vi "ChangePlotSize.vi"(8 "error in (no error)":errorcluster caption="错误输入（无错误）", 11 "TPlot 输入":refnum<class "TPlot.lvclass">) -> (0 "error out":errorcluster caption="错误输出", 3 "TPlot 输出":refnum<class "TPlot.lvclass">)   [LabVIEW 2018, in "DataDisplay.lvlib" / "TPlot.lvclass"]
uses:
  TPlot.lvclass
  <vilib>/Utility/miscctls.llb/LVBoundsTypeDef.ctl
  <vilib>/Utility/miscctls.llb/LVPositionTypeDef.ctl
  TPlot.lvclass/TPlot.ctl
panel:
  out "波形图":waveform(dbl)[](graph)
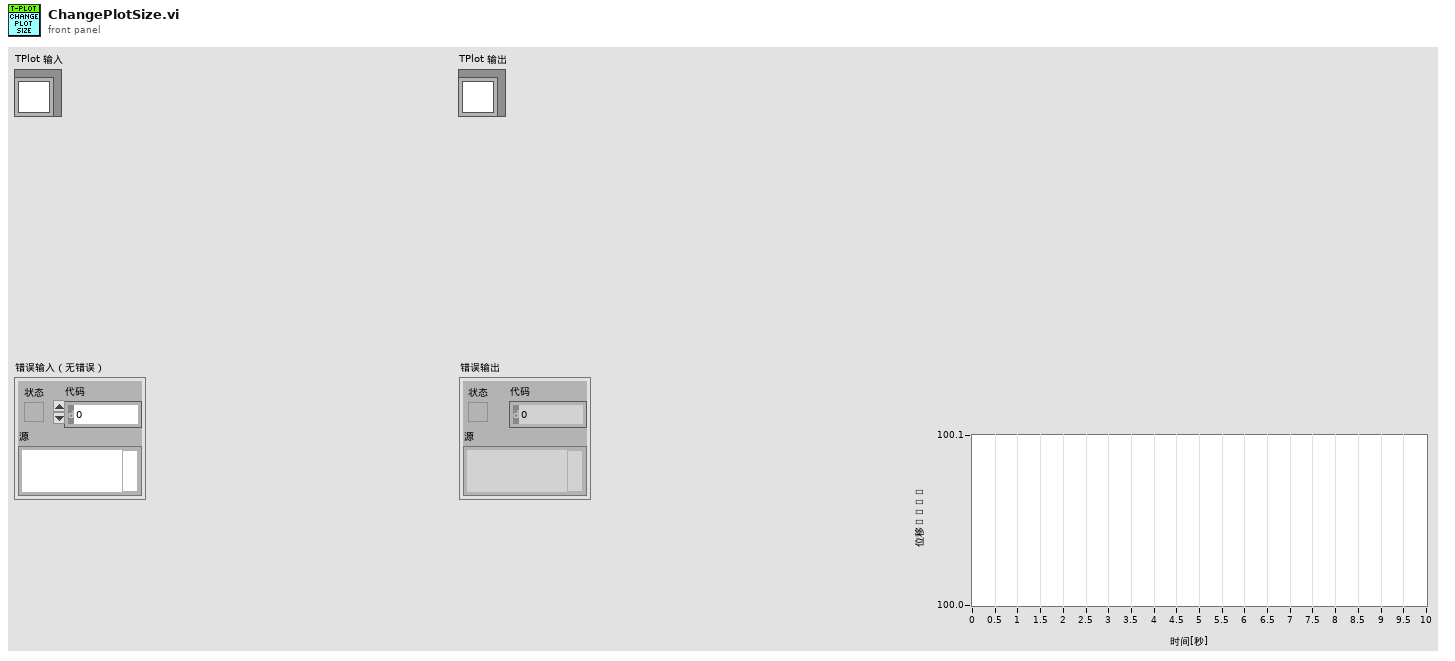
[diagram p1: front panel]
types:
  T1 = typedef "LVPositionTypeDef.ctl" = cluster{"Left":i32, "Top":i32}
  T2 = typedef "LVBoundsTypeDef.ctl" = cluster{"Width":u32, "Height":u32}
  T3 = typedef "LVRectTypeDef.ctl" = cluster{"Left":i16, "Top":i16, "Right":i16, "Bottom":i16}
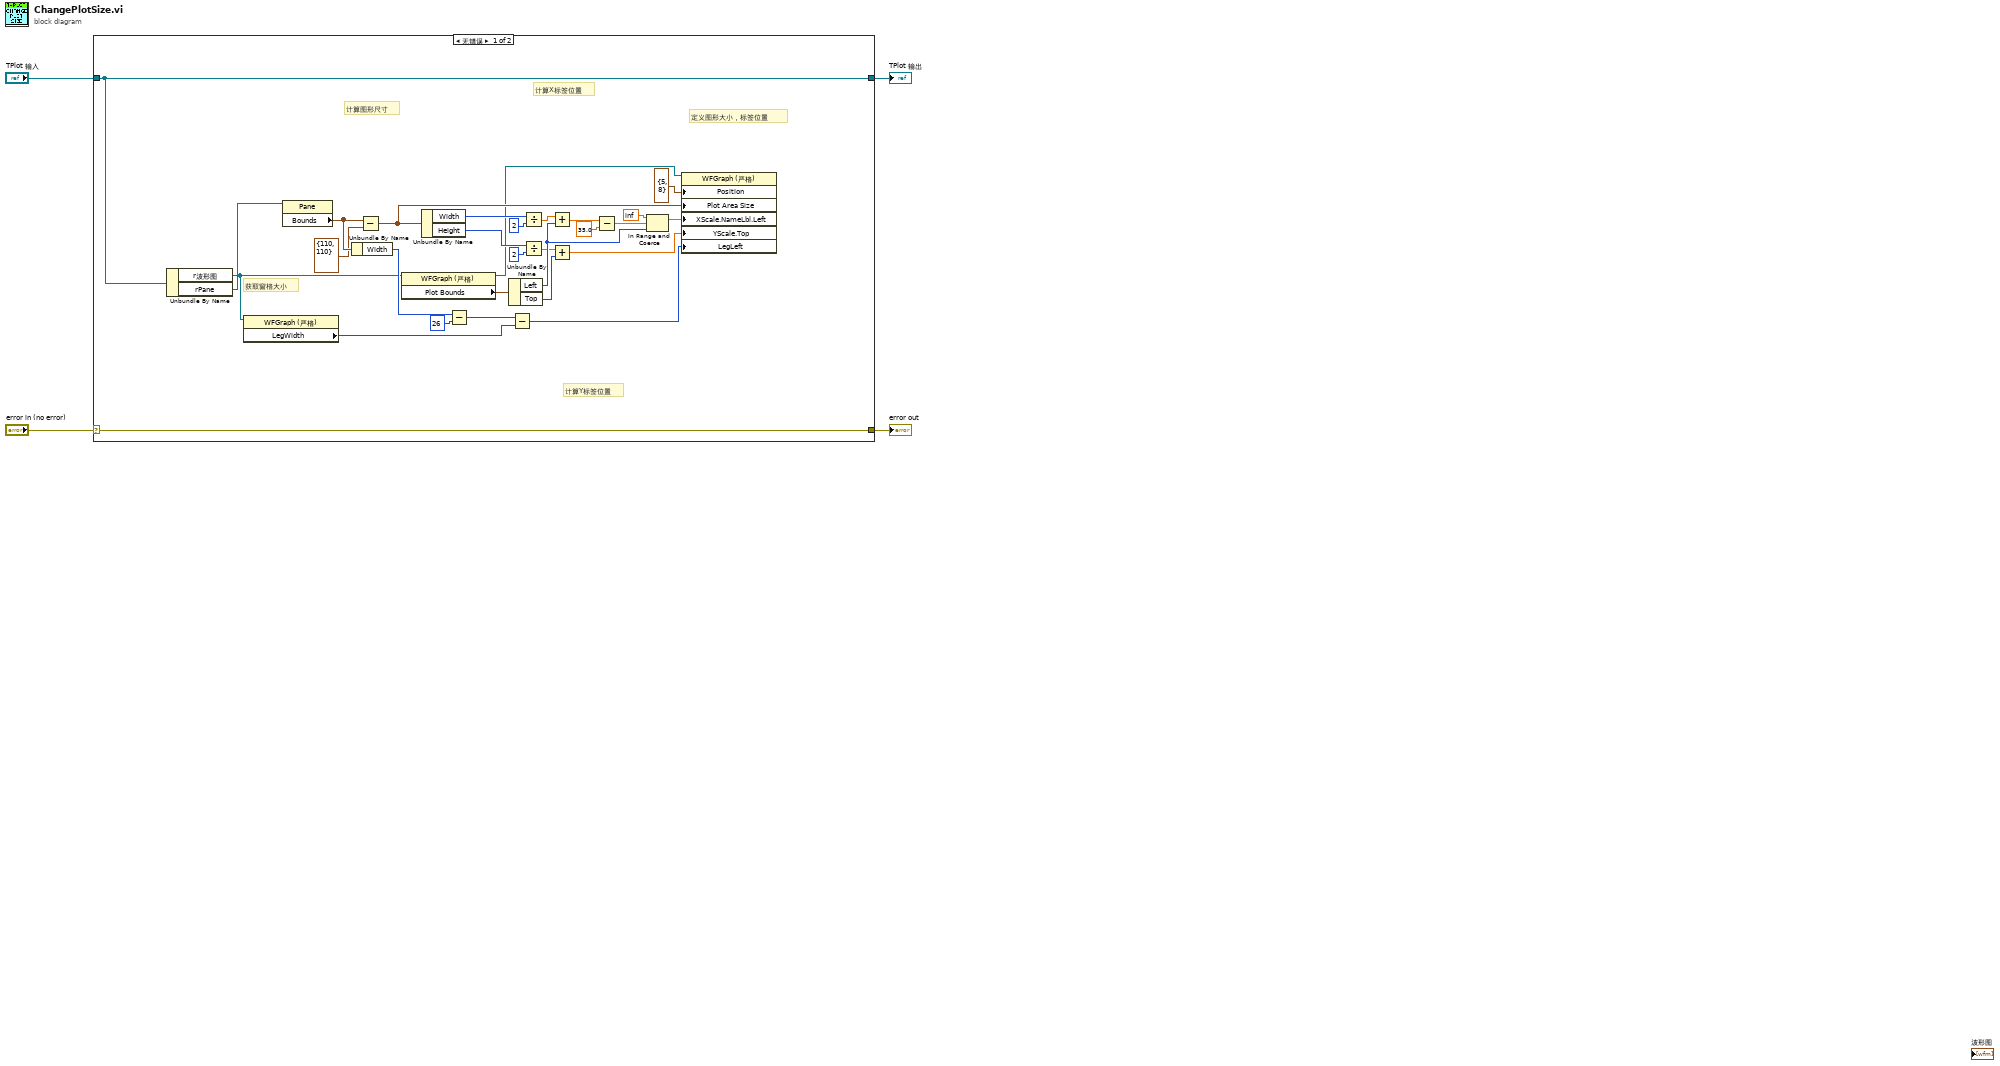
[diagram p0: block diagram]
diagram:
  n1 = case shown="无错误" "error in (no error)" {
    selector: "error in (no error)" -> [w33 w35]
    tunnel: [w33 w35] -> w3
    tunnel: [w10 w34] -> w1
    tunnel: "TPlot 输入" -> [w10 w34]
    frame No Error {
      # "定义图形大小，标签位置"
      # "计算X标签位置"
      # "计算Y标签位置"
      # "计算图形尺寸"
      # "获取窗格大小"
      n2 = Unbundle By Name(w10) -> ("r波形图"=w7:refnum<vi>, "rPane"=w8:refnum<vi>)
      n3 = property class="WFGraph (严格)"(reference=w7) -> ("LegWidth"=w26:u32)  [unwired: 1 in, 2 out]
      n4 = property class="Pane"(reference=w8) -> ("Bounds"=w27:T2)  [unwired: 1 in, 2 out]
      n5 = Unbundle By Name(w27) -> ("Width"=w24:u32)
      n6 = Subtract(x=w27, y=T2 {"Width"=110, "Height"=110}) -> (x-y=w23:T2)
      n7 = property class="WFGraph (严格)"(reference=w7) -> (reference out=w15:refnum<vi>, "Plot Bounds"=w19:T3)  [unwired: 1 in, 1 out]
      n8 = Unbundle By Name(w23) -> ("Width"=w20:u32, "Height"=w22:u32)
      n9 = Subtract(x=w24, y=u32 26) -> (x-y=w25:u32)
      n10 = Unbundle By Name(w19) -> ("Left"=w30:i16, "Top"=w21:i16)
      n11 = Subtract(x=w25, y=w26) -> (x-y=w28:u32)
      n12 = Divide(x=w20, y=u32 2) -> (x/y=w16:dbl)
      n13 = Divide(x=w22, y=u32 2) -> (x/y=w17:dbl)
      n14 = Add(x=w16, y=w30) -> (x+y=w29:dbl)
      n15 = Add(x=w17, y=w21) -> (x+y=w18:dbl)
      n16 = Subtract(x=w29, y=35.0) -> (x-y=w31:dbl)
      n17 = In Range and Coerce(upper limit=inf, x=w31, lower limit=w30) -> (coerced(x)=w32:dbl)  [unwired: 1 out]
      n18 = property class="WFGraph (严格)"(reference=w15, "Position"=T1 {"Left"=5, "Top"=8} ("位置"), "Plot Area Size"=w23, "XScale.NameLbl.Left"=w32, "YScale.Top"=w18, "LegLeft"=w28) -> ()  [unwired: 1 in, 2 out]
    }
    frame Error {
    }
  }
  "error out" <- w3
  "TPlot 输出" <- w1
